vi "SR7265 Write DAQs.vi"(8 "Error In":errorcluster, 10 "Data":dbl[](array[numeric]), 11 "VISA resource":refnum<visa-resource-name>) -> (0 "Error Out":errorcluster, 3 "VISA resource dup":refnum<visa-resource-name>)   [LabVIEW 2019]
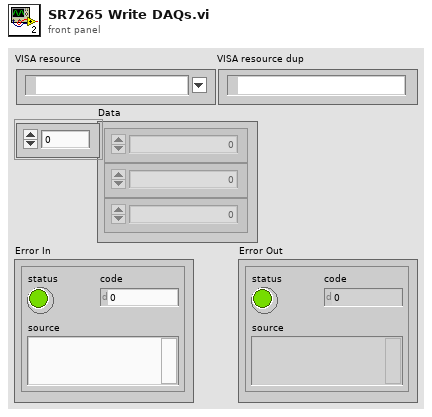
[diagram p1: front panel]
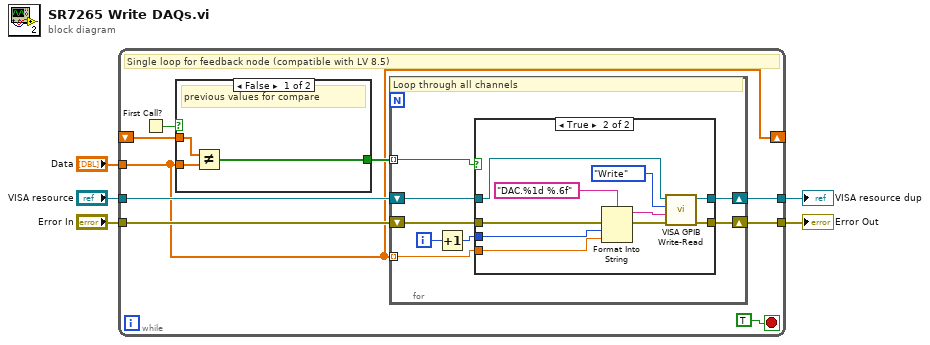
[diagram p0: block diagram]
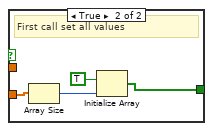
[diagram p2: hidden frame]
diagram:
  n1 = while {
    tunnel: [w9] -> w5
    tunnel: [w8] -> w4
    tunnel: "VISA resource" -> [w13]
    tunnel: "Error In" -> [w12]
    shift-right: [w7] -> _
    shift-left: _ -> [w6]
    tunnel: "Data" -> [w7]
    stop <- TRUE stop-if-true
    # "Single loop for feedback node (compatible with LV 8.5)"
    n2 = First Call?() -> (First Call?: T/F=w11:bool)
    n3 = case shown="False" w11 {
      tunnel: w7 -> [w16 w19]
      tunnel: [w17 w18] -> w10
      tunnel: w6 -> [w15 _]
      frame False {
        # "previous values for compare"
        n4 = Not Equal?(x=w15, y=w16) -> (x != y?=w17:bool[])
      }
      frame True {
        # "First call set all values"
        n5 = Array Size(array=w19) -> (size(s)=w21:i32)
        n6 = Initialize Array(TRUE, w21) -> (w18:bool[])
      }
    }
    n7 = for {
      tunnel: w10 -> [w28] mode=indexing
      tunnel: w7 -> [w27] mode=indexing
      shift-right: [w23] -> w9
      shift-left: w13 -> [w25]
      shift-right: [w22] -> w8
      shift-left: w12 -> [w24]
      i -> [w29]
      # "Loop through all channels"
      n8 = Increment(x=w29) -> (x+1=w26:i32)
      n9 = case shown="True" w28 {
        tunnel: w27 -> [_ w40]
        tunnel: w26 -> [_ w39]
        tunnel: [w31 w34] -> w23
        tunnel: w25 -> [w31 w36]
        tunnel: [w30 w32] -> w22
        tunnel: w24 -> [w30 w35]
        frame False {
        }
        frame True {
          n10 = Format Into String(format string="DAC.%1d %.6f", error in=w35, w39, w40) -> (resulting string=w37:string, error out=w33:errorcluster)  [unwired: 1 in]
          n11 = call "VISA GPIB Write-Read.vi"("error in (no error)"=w33, "Command"=w37, "Action"=enum16{"Write", "Read", "Write & Read"}."Write", "VISA resource name"=w36) -> ("error out"=w32:errorcluster, "dup VISA Session"=w34:refnum<visa-resource-name>)  [unwired: 4 in, 2 out]
        }
      }
    }
  }
  "VISA resource dup" <- w5
  "Error Out" <- w4
